vi "Get Curve Data.vi"(0 "VISA session":refnum<visa-resource-name>, 1 "Curve #":i32, 2 "error in (no error)":errorcluster) -> (3 "dup VISA session":refnum<visa-resource-name>, 4 "Temperature":dbl[](array[numeric]) format="%.3e", 5 "Resistance":dbl[](array[numeric]) format="%.3e", 6 "error out":errorcluster)   [LabVIEW 2019]
doc: "This VI will download and graph a calibration curve from a LakeShore Model 370 AC Resistance Bridge.\nScott Hannahs, <sth@magnet.fsu.edu> NHMFL-FSU, May 2003"
panel:
  out "# of Points":i32
  out "XY Graph":cluster{dbl[], dbl[]}(graph)
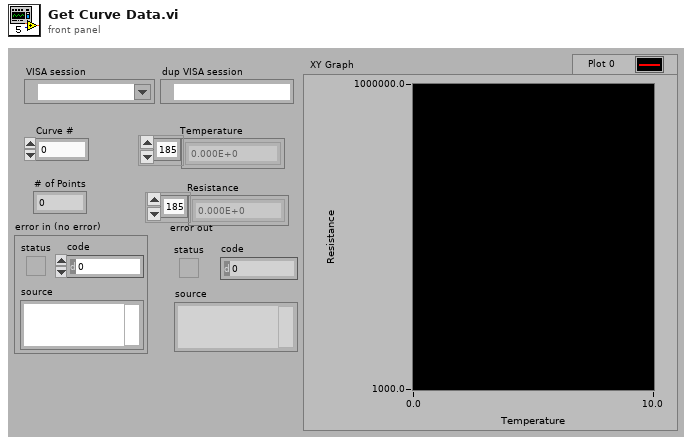
[diagram p1: front panel]
types:
  T1 = typedef "Data Format.ctl" = u16
  T2 = cluster{"Curve ID":string, "Serial Number":string, "Data Format":T1, "Setpoint Limit":dbl, "Temp. Coef":u16}
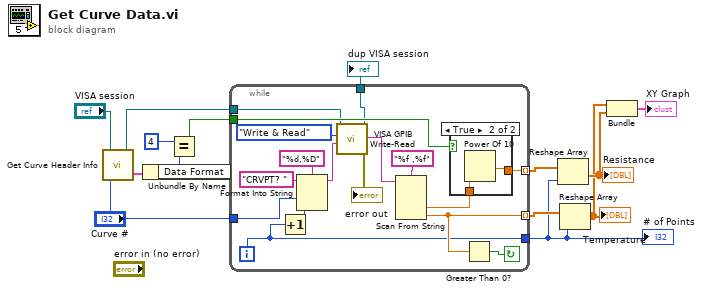
[diagram p0: block diagram]
diagram:
  n1 = call "Get Curve Header Info.vi"("Curve #"="Curve #", "VISA session"="VISA session") -> ("Cluster"=w9:T2, "dup VISA session"=w12:refnum<visa-resource-name>)
  n2 = Unbundle By Name(w9) -> ("Data Format"=w8:T1)
  n3 = Equal?(x=u16 4, y=w8) -> (x = y?=w6:bool)
  n4 = while {
    tunnel: [w22] -> w14 mode=indexing
    tunnel: [w20] -> w13 mode=indexing
    tunnel: w12 -> [w16]
    tunnel: "Curve #" -> [w25]
    tunnel: w6 -> [w24]
    tunnel: [w18] -> w5
    tunnel: [w15] -> w1
    i -> [w18]
    stop <- w21 continue-if-true
    n5 = Increment(x=w18) -> (x+1=w19:i32)
    n6 = Format Into String(format string="%d,%D", initial string="CRVPT? " ("String to Write"), w25, w19) -> (resulting string=w30:string)  [unwired: 1 in, 1 out]
    n7 = call "VISA GPIB Write-Read.vi"("Command"=w30, "Action"=enum16{"Write", "Read", "Write & Read"}."Write & Read", "VISA resource name"=w16) -> ("error out"=→"error out":errorcluster, "String Returned"=w26:string, "dup VISA Session"=w15:refnum<visa-resource-name>)  [unwired: 5 in, 1 out]
    n8 = Scan From String(format string="%f ,%f", input string=w26) -> (output 1=w23:dbl, output 2=w20:dbl)  [unwired: 4 in, 3 out]
    n9 = case shown="True" w24 {
      tunnel: w23 -> [w32 w34]
      tunnel: [w32 w33] -> w22
      frame False {
      }
      frame True {
        n10 = Power Of 10(x=w34) -> (10^x=w33:dbl)
      }
    }
    n11 = Greater Than 0?(x=w20) -> (x > 0?=w21:bool)
  }
  "dup VISA session" <- w1
  "# of Points" <- w5
  n12 = Reshape Array(w14, w5) -> (w3:dbl[])
  "Resistance" <- w3
  n13 = Reshape Array(w13, w5) -> (w2:dbl[])
  "Temperature" <- w2
  n14 = Bundle(w2, w3) -> (→"XY Graph":cluster{dbl[], dbl[]})  [unwired: 1 in]
